vi "HeaderCondenser.vi"(0 "Consumer P/N":string, 3 "GeneralResult":string, 5 "P/N UUT":string, 7 "ApprovedBy":string, 9 "Driver S/N":string, 11 "error in":errorcluster, 12 "Parameters Ver.":string, 13 "Oper.":string, 14 "Tester Software Ver":string) -> (6 "Array":string[][](array[string]), 15 "error out":errorcluster)   [LabVIEW 2017]
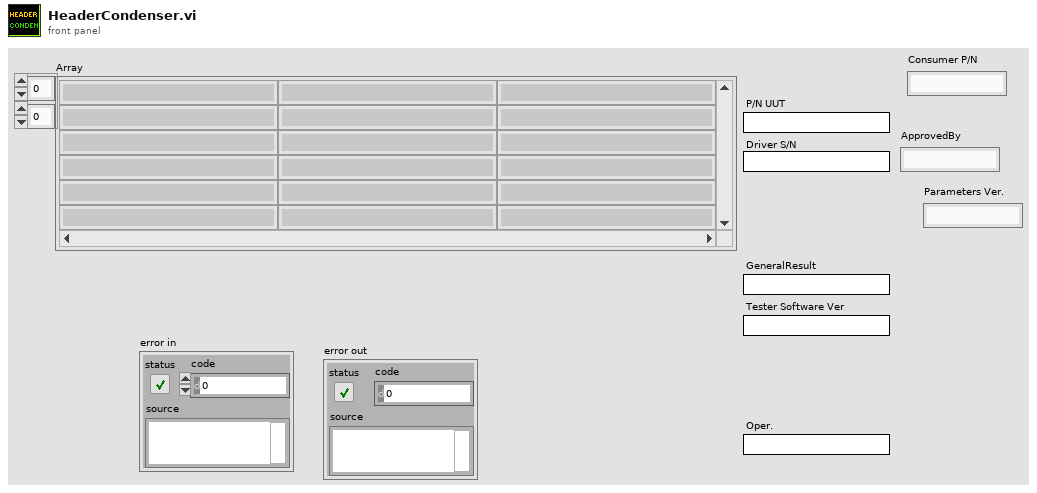
[diagram p1: front panel]
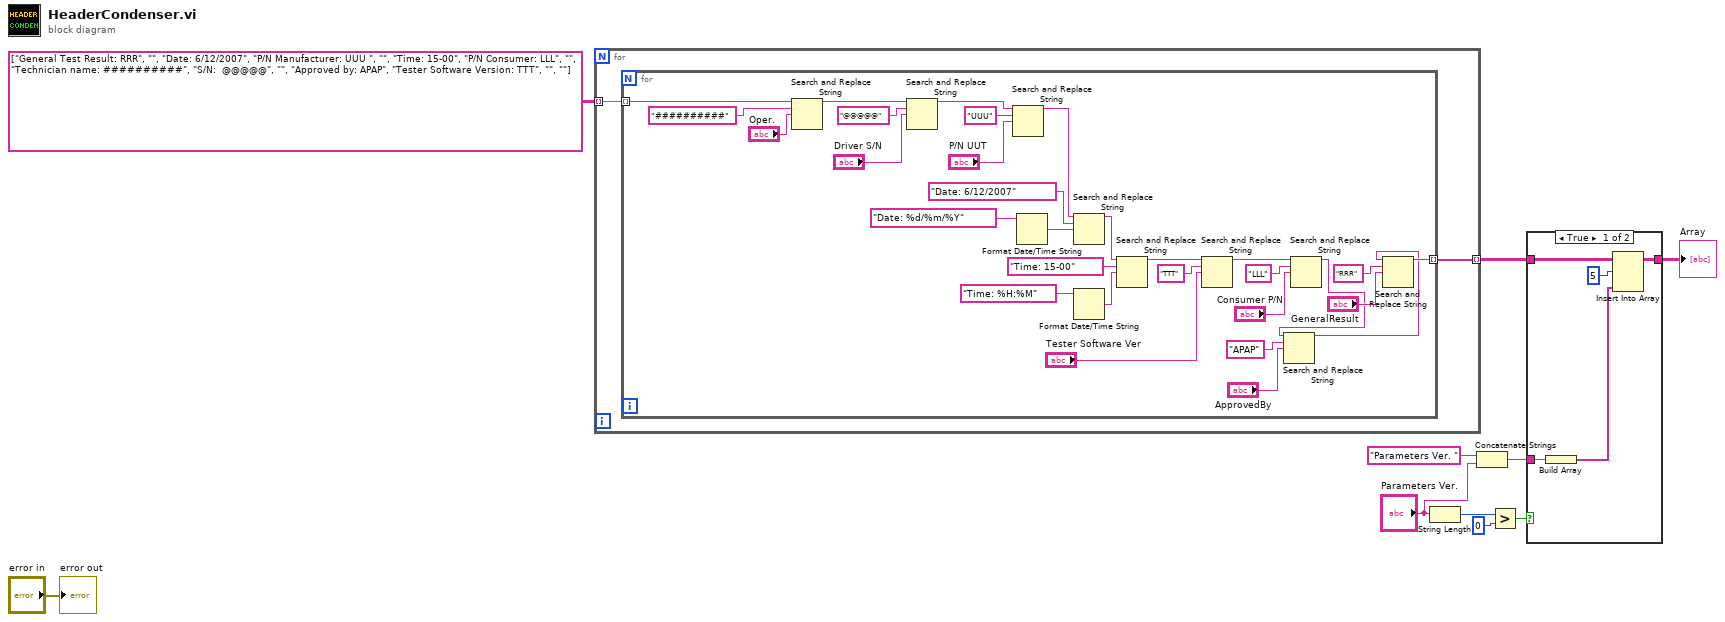
[diagram p0: block diagram]
diagram:
  n1 = for {
    tunnel: string[][] [["General Test Result: RRR", "", "Date: 6/12/2007"], ["P/N Manufacturer: UUU ", "", "Time: 15-00"], ["P/N Consumer: LLL", "", "Technician name: ##########"], ["S/N:  @@@@@", "", "Approved by: APAP"], ["Tester Software Version: TTT", "", ""]] -> [w12] mode=indexing
    tunnel: [w11] -> w6 mode=indexing
    n2 = for {
      tunnel: w12 -> [w21] mode=indexing
      tunnel: [w20] -> w11 mode=indexing
      n3 = Search and Replace String(input string=w21, search string="##########" ("source"), replace string="Oper.") -> (result string=w32:string)  [unwired: 5 in, 3 out]
      n4 = Search and Replace String(input string=w32, search string="@@@@@" ("source"), replace string="Driver S/N") -> (result string=w34:string)  [unwired: 5 in, 3 out]
      n5 = Search and Replace String(input string=w34, search string="UUU" ("source"), replace string="P/N UUT") -> (result string=w33:string)  [unwired: 5 in, 3 out]
      n6 = Format Date/Time String(time format string (%c)="Date: %d/%m/%Y") -> (date/time string=w31:string)  [unwired: 2 in]
      n7 = Search and Replace String(input string=w33, search string="Date: 6/12/2007" ("time format string (%c)"), replace string=w31) -> (result string=w39:string)  [unwired: 5 in, 3 out]
      n8 = Format Date/Time String(time format string (%c)="Time: %H:%M") -> (date/time string=w41:string)  [unwired: 2 in]
      n9 = Search and Replace String(input string=w39, search string="Time: 15-00", replace string=w41) -> (result string=w40:string)  [unwired: 5 in, 3 out]
      n10 = Search and Replace String(input string=w40, search string="TTT", replace string="Tester Software Ver") -> (result string=w19:string)  [unwired: 5 in, 3 out]
      n11 = Search and Replace String(input string=w19, search string="LLL", replace string="Consumer P/N") -> (result string=w14:string)  [unwired: 5 in, 3 out]
      n12 = Search and Replace String(input string=w14, search string="APAP", replace string="ApprovedBy") -> (result string=w13:string)  [unwired: 5 in, 3 out]
      n13 = Search and Replace String(input string=w13, search string="RRR", replace string="GeneralResult") -> (result string=w20:string)  [unwired: 5 in, 3 out]
    }
  }
  n14 = String Length(string="Parameters Ver.") -> (length=w3:i32)
  n15 = Concatenate Strings("Parameters Ver. " ("string"), "Parameters Ver.") -> (w4:string)
  n16 = Greater?(x=w3, y=0) -> (0:w1:bool)
  n17 = case shown="True" w1 {
    tunnel: w6 -> [w47 w48]
    tunnel: [w43 w48] -> w5
    tunnel: w4 -> [w45 _]
    frame True {
      n18 = Build Array(w45) -> (w44:string[])
      n19 = Insert Into Array(array=w47, index (row)=5, new element=w44) -> (w43:string[][])  [unwired: 1 in]
    }
    frame False {
    }
  }
  "Array" <- w5
  "error out" <- "error in"
